vi "Vision Processing.vi"(4 "error in (no error)":errorcluster, 7 "Image Size 0":T1=enum."320x240") -> ()   [LabVIEW 2016]
doc: "This VI runs in parallel to other tasks. It gets images from the camera, processes them for color or shape and use that information to affect robot behavior."
uses:
  <vilib>/Rock Robotics/WPI/Camera/WPI_CameraImageSize.ctl
  <vilib>/Rock Robotics/WPI/Camera/WPI_CameraExposure Values.ctl
  <vilib>/Rock Robotics/WPI/Camera/WPI_CameraFrameRate.ctl
  <vilib>/Rock Robotics/WPI/Camera/WPI_CameraWhite Balance Values.ctl
  Refname/Cameras.ctl
  Robot Global Data.vi
  Refname/Refname to String (Cameras).vi
  <vilib>/Rock Robotics/Network Tables/NT Write String.vi
panel:
  in  "Image Size 1":T1=enum."320x240"
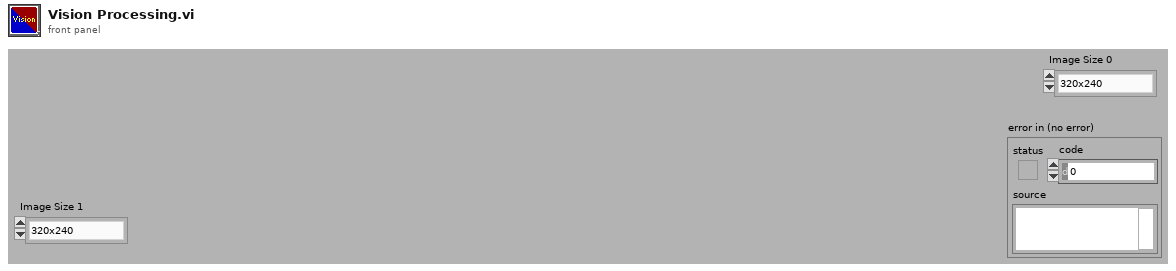
[diagram p1: front panel]
types:
  T1 = typedef "WPI_CameraImageSize.ctl" = enum16{"640x480", "320x240", "160x120", "Custom"}
  T2 = typedef "WPI_CameraWhite Balance Values.ctl" = enum16{"Auto", "Fixed indoor", "Fixed outdoor 1", "Fixed outdoor 2", "Fixed fluorescent 1", "Fixed fluorescent 2", "Hold current", "Custom"}
  T3 = typedef "WPI_CameraFrameRate.ctl" = u32
  T4 = typedef "WPI_CameraExposure Values.ctl" = enum16{"Auto", "Flicker-free 50 Hz", "Flicker-free 60 Hz", "Hold current", "Custom"}
  T5 = typedef "Image Type" = u32
  T6 = typedef "WPI_CameraDevRef.ctl" = cluster{"Camera Address":string, "CameraStatus":errorcluster}
  T7 = typedef "IMAQ Image.ctl" = refnum<image>
  T8 = typedef "Cameras.ctl" = enum16{"Gear", "Climber"}
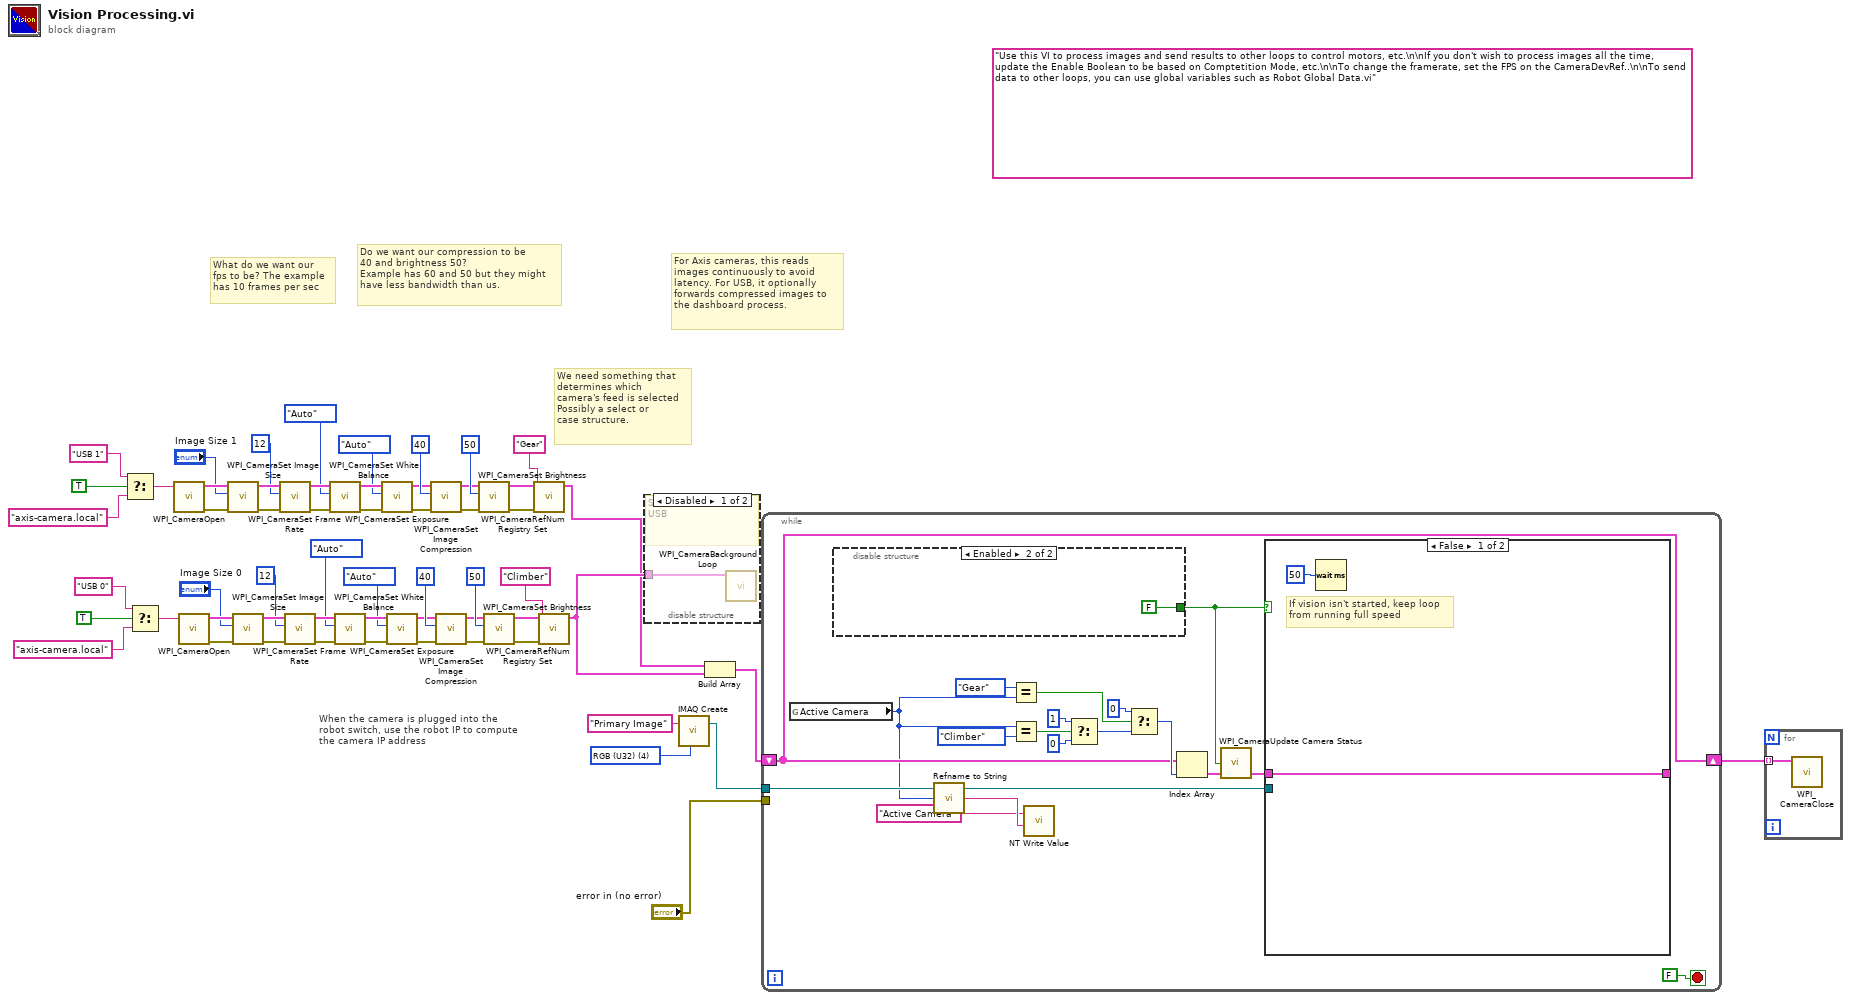
[diagram p0: block diagram]
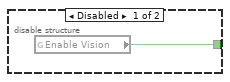
[diagram p3: hidden frame]
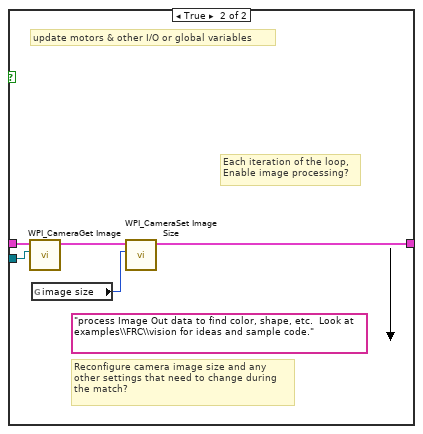
[diagram p4: hidden frame]
diagram:
  (unwired) "Use this VI to process images and send results to other loops to control motors, etc.\n\nIf you don't wish to process images all the time, update the Enable Boolean to be based on Comptetition Mode, etc.\n\nTo change the framerate, set the FPS on the CameraDevRef..\n\nTo send data to other loops, you can use global variables such as Robot Global Data.vi"
  w58 = T5 4 items=["Grayscale (U8)", "Grayscale (I16)", "Grayscale (SGL)", "Complex (CSG)", "RGB (U32)", "HSL (U32)", "RGB (U64)"] ("Image Type")
  # "We need something that \ndetermines which \ncamera's feed is selected \nPossibly a select or \ncase structure."
  # "Do we want our compression to be\n40 and brightness 50?\nExample has 60 and 50 but they might\nhave less bandwidth than us."
  # "What do we want our\nfps to be? The example\nhas 10 frames per sec"
  # "When the camera is plugged into the\nrobot switch, use the robot IP to compute\nthe camera IP address"
  # "For Axis cameras, this reads\nimages continuously to avoid\nlatency. For USB, it optionally\nforwards compressed images to\nthe dashboard process."
  n1 = Select(t="USB 1" ("format string"), s=TRUE ("dot notation? (F)"), f="axis-camera.local" ("format string")) -> (s? t:f=w6:string)
  n2 = Select(t="USB 0" ("format string"), s=TRUE ("dot notation? (F)"), f="axis-camera.local" ("format string")) -> (s? t:f=w31:string)
  n3 = call <vilib>:"WPI_CameraOpen.vi"("Camera Address"=w6) -> ("error out"=w20:errorcluster, "CameraDevRef"=w21:T6)  [unwired: 1 in, 8 out]
  n4 = call <vilib>:"WPI_CameraOpen.vi"("Camera Address"=w31) -> ("error out"=w46:errorcluster, "CameraDevRef"=w47:T6)  [unwired: 1 in, 8 out]
  n5 = call <vilib>:"WPI_CameraSet Image Size.vi"("error in (no error)"=w20, "Image Size"="Image Size 1", "CameraDevRef"=w21) -> ("error out"=w19:errorcluster, "CameraDevRef Out"=w22:T6)  [unwired: 1 in, 6 out]
  n6 = call <vilib>:"WPI_CameraSet Image Size.vi"("error in (no error)"=w46, "Image Size"="Image Size 0", "CameraDevRef"=w47) -> ("error out"=w45:errorcluster, "CameraDevRef Out"=w48:T6)  [unwired: 1 in, 6 out]
  n7 = call <vilib>:"WPI_CameraSet Frame Rate.vi"("error in (no error)"=w19, "Frame Rate (fps)"=T3 12, "CameraDevRef"=w22) -> ("error out"=w18:errorcluster, "CameraDevRef Out"=w24:T6)  [unwired: 7 out]
  n8 = call <vilib>:"WPI_CameraSet Frame Rate.vi"("error in (no error)"=w45, "Frame Rate (fps)"=T3 12, "CameraDevRef"=w48) -> ("error out"=w44:errorcluster, "CameraDevRef Out"=w50:T6)  [unwired: 7 out]
  n9 = call <vilib>:"WPI_CameraSet White Balance.vi"("error in (no error)"=w18, "White Balance"=WPI_CameraWhite_Balance_Values."Auto", "CameraDevRef"=w24) -> ("error out"=w17:errorcluster, "CameraDevRef Out"=w23:T6)  [unwired: 1 in, 6 out]
  n10 = call <vilib>:"WPI_CameraSet White Balance.vi"("error in (no error)"=w44, "White Balance"=WPI_CameraWhite_Balance_Values."Auto", "CameraDevRef"=w50) -> ("error out"=w43:errorcluster, "CameraDevRef Out"=w49:T6)  [unwired: 1 in, 6 out]
  n11 = call <vilib>:"WPI_CameraSet Exposure.vi"("error in (no error)"=w17, "Exposure"=WPI_CameraExposure_Values."Auto", "CameraDevRef"=w23) -> ("error out"=w16:errorcluster, "CameraDevRef Out"=w26:T6)  [unwired: 1 in, 6 out]
  n12 = call <vilib>:"WPI_CameraSet Exposure.vi"("error in (no error)"=w43, "Exposure"=WPI_CameraExposure_Values."Auto", "CameraDevRef"=w49) -> ("error out"=w42:errorcluster, "CameraDevRef Out"=w52:T6)  [unwired: 1 in, 6 out]
  n13 = call <vilib>:"WPI_CameraSet Image Compression.vi"("error in (no error)"=w16, "Compression"=40, "CameraDevRef"=w26) -> ("error out"=w15:errorcluster, "CameraDevRef Out"=w25:T6)  [unwired: 7 out]
  n14 = call <vilib>:"WPI_CameraSet Image Compression.vi"("error in (no error)"=w42, "Compression"=40, "CameraDevRef"=w52) -> ("error out"=w41:errorcluster, "CameraDevRef Out"=w51:T6)  [unwired: 7 out]
  n15 = call <vilib>:"WPI_CameraSet Brightness.vi"("error in (no error)"=w15, "Brightness"=50, "CameraDevRef"=w25) -> ("error out"=w13:errorcluster, "CameraDevRef Out"=w14:T6)  [unwired: 7 out]
  n16 = call <vilib>:"WPI_CameraSet Brightness.vi"("error in (no error)"=w41, "Brightness"=50, "CameraDevRef"=w51) -> ("error out"=w39:errorcluster, "CameraDevRef Out"=w40:T6)  [unwired: 7 out]
  n17 = call <vilib>:"WPI_CameraRefNum Registry Set.vi"("error in (no error)"=w13, "refnum name"="Gear", "CameraDevRef"=w14) -> ("CameraDevRef"=w3:T6)  [unwired: 1 in, 7 out]
  n18 = call <vilib>:"WPI_CameraRefNum Registry Set.vi"("error in (no error)"=w39, "refnum name"="Climber", "CameraDevRef"=w40) -> ("CameraDevRef"=w4:T6)  [unwired: 1 in, 7 out]
  n19 = disable-structure shown="Disabled" {
    disable-tunnel: w4 -> [w59 _]
    frame Disabled {
      # "Seems useless for USB"
      n20 = call <vilib>:"WPI_CameraBackground Loop.vi"("CameraDevRef"=w59) -> ()  [unwired: 11 in]
    }
    frame Enabled {
    }
  }
  n21 = call "IMAQ Create"("Image Name"="Primary Image", "Image Type"=w58) -> ("New Image"=w56:T7)  [unwired: 2 in, 2 out]
  n22 = Build Array(w3, w4) -> (w2:T6[])
  n23 = while {
    shift-right: [w63] -> w1
    shift-left: w2 -> [w63]
    tunnel: w56 -> [w76]
    tunnel: "error in (no error)" -> [_]
    stop <- FALSE stop-if-true
    n24 = global read "Robot Global Data.vi" "Active Camera"() -> (w62:T8)
    n25 = disable-structure shown="Enabled" {
      disable-tunnel: [w78 FALSE ("Enable Vision")] -> w74
      frame Disabled {
        n26 = global read "Robot Global Data.vi" "Enable Vision"() -> (w78:bool)
      }
      frame Enabled {
      }
    }
    n27 = call-poly "Refname to String.vi"("Enum"=w62) -> ("String"=w61:string)
    n28 = Equal?(x=Cameras."Gear", y=w62) -> (x = y?=w71:bool)
    n29 = Equal?(x=w62, y=Cameras."Climber") -> (x = y?=w67:bool)
    n30 = call-poly <vilib>:"NT Write Value.vi"("String"=w61, "Name"="Active Camera") -> ()  [unwired: 9 in, 1 out]
    n31 = Select(t=1, s=w67, f=0) -> (s? t:f=w65:i32)
    n32 = Select(t=0, s=w71, f=w65) -> (s? t:f=w69:i32)
    n33 = Index Array(array=w63, index=w69) -> (element=w73:T6)
    n34 = call <vilib>:"WPI_CameraUpdate Camera Status.vi"("CameraDevRef In"=w73, "Enable Vision"=w74) -> ("CameraDevRef Out"=w75:T6)  [unwired: 3 in]
    n35 = case shown="False" w74 {
      tunnel: w76 -> [_ w85]
      tunnel: [w81 w86] -> _
      tunnel: w75 -> [w81 w83]
      frame False {
        # "If vision isn't started, keep loop\nfrom running full speed"
        n36 = Wait (ms)(milliseconds to wait=u32 50) -> ()  [unwired: 1 out]
      }
      frame True {
        (unwired) "process Image Out data to find color, shape, etc.  Look at examples\\FRC\\vision for ideas and sample code."
        # "Each iteration of the loop,\nEnable image processing?"
        # "update motors & other I/O or global variables"
        # "Reconfigure camera image size and any\nother settings that need to change during\nthe match?"
        n37 = call <vilib>:"WPI_CameraGet Image.vi"("Image"=w85, "CameraDevRef"=w83) -> ("CameraDevRef Out"=w82:T6)  [unwired: 1 in, 8 out]
        n38 = global read "Robot Global Data.vi" "image size"() -> (w84:T1)
        n39 = call <vilib>:"WPI_CameraSet Image Size.vi"("Image Size"=w84, "CameraDevRef"=w82) -> ("CameraDevRef Out"=w86:T6)  [unwired: 2 in, 7 out]
      }
    }
  }
  n40 = for {
    tunnel: w1 -> [w87] mode=indexing
    n41 = call <vilib>:"WPI_CameraClose.vi"("CameraDevRef"=w87) -> ()  [unwired: 1 in, 10 out]
  }
